vi "combosToRanges.vi"(11 "combosIn":T1[][](array[typedef])) -> (3 "rangesOut":T3[](array[typedef]))   [LabVIEW 2016]
uses:
  ComboRange.ctl
  MFCdescription.ctl
  MFCcapability.ctl
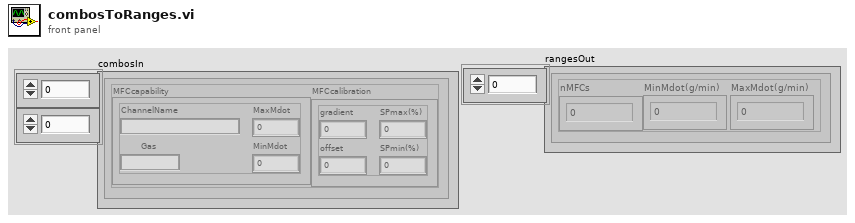
[diagram p1: front panel]
types:
  T1 = typedef "MFCdescription.ctl" = cluster{"MFCcapability":T2, "MFCcalibration":cluster{"gradient":dbl, "offset":dbl, "SPmin(%)":dbl, "SPmax(%)":dbl}}
  T2 = typedef "MFCcapability.ctl" = cluster{"ChannelName":string, "MinMdot":dbl, "MaxMdot":dbl, "Gas":string}
  T3 = typedef "ComboRange.ctl" = cluster{"nMFCs":i32, "MinMdot(g/min)":dbl, "MaxMdot(g/min)":dbl}
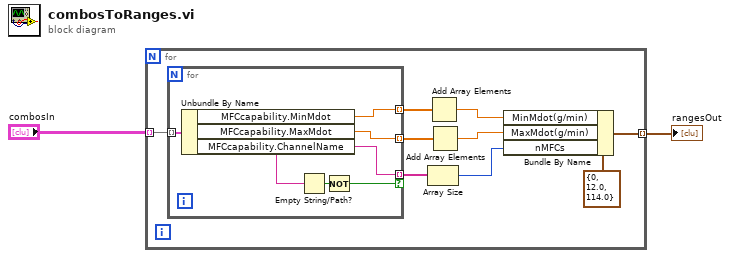
[diagram p0: block diagram]
diagram:
  n1 = for {
    tunnel: "combosIn" -> [w9] mode=indexing
    tunnel: [w3] -> w2 mode=indexing
    n2 = for {
      tunnel: [w16] -> w11 mode=indexing
      tunnel: [w15] -> w10 mode=indexing if=w12
      tunnel: w9 -> [w14] mode=indexing
      tunnel: [w13] -> w8 mode=indexing
      n3 = Unbundle By Name(w14) -> ("MFCcapability.MinMdot"=w13:dbl, "MFCcapability.MaxMdot"=w16:dbl, "MFCcapability.ChannelName"=w15:string)
      n4 = Empty String/Path?(string/path=w15) -> (empty?=w17:bool)
      n5 = Not(x=w17) -> (.not. x?=w12:bool)
    }
    n6 = Array Size(array=w10) -> (size(s)=w4:i32)
    n7 = Add Array Elements(numeric array=w8) -> (sum=w6:dbl)
    n8 = Add Array Elements(numeric array=w11) -> (sum=w5:dbl)
    n9 = Bundle By Name(cluster=T3 {"nMFCs"=0, "MinMdot(g/min)"=12.0, "MaxMdot(g/min)"=114.0} ("Cluster"), "MinMdot(g/min)"=w6, "MaxMdot(g/min)"=w5, "nMFCs"=w4) -> (w3:T3)
  }
  "rangesOut" <- w2
